vi "Accelerometer Display.vi"(1 "Accel Range":T2, 2 "Mode":enum8{"Start", "Run", "Finish"}(ring)) -> (0 "Distances":cluster{"X":dbl, "Y":dbl, "Z":dbl})   [LabVIEW 2014]
uses:
  <vilib>/Rock Robotics/WPI/Accelerometer/WPI_AccelerometerRange.ctl
  <vilib>/Rock Robotics/WPI/Accelerometer/InternalAccelerometer/WPI_AccelerometerInternalOpen.vi
  <vilib>/Analysis/NI_AALPro.lvlib
panel:
  out "Y Distance 2":dbl(graph)
  out "Z Distance":dbl(graph)
  out "Y Distance":dbl(graph)
  out "Waveform Chart":T1(graph)
  out "Z Acceleration":dbl
  out "Y Acceleration":dbl
  out "X Acceleration":dbl
  # "Set these inputs before running."
  # "Output information"
  # "This uses the internal accelerometer built into the roboRIO.  No wiring is necessary."
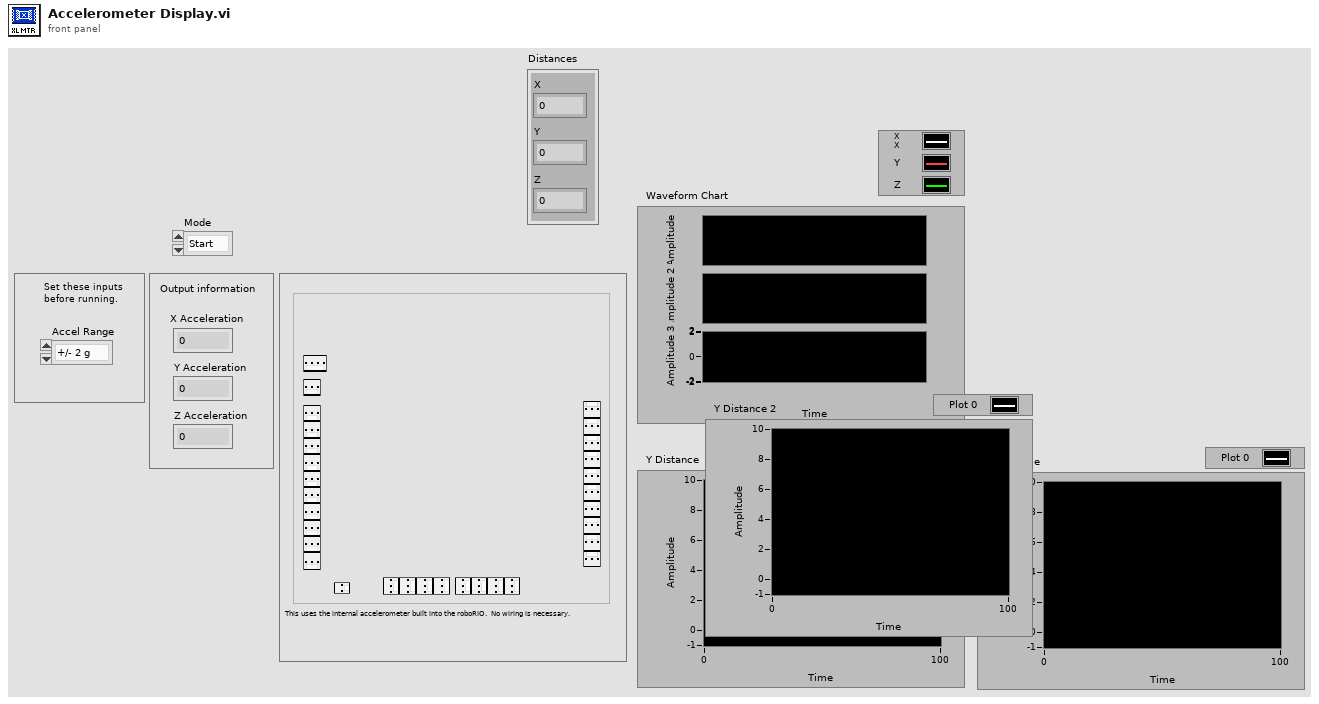
[diagram p1: front panel]
types:
  T1 = cluster{"X-Axis":dbl, "Y-Axis":dbl, "Z-Axis":dbl}
  T2 = typedef "WPI_AccelerometerRange.ctl" = enum16{"+/- 2 g", "+/- 4 g", "+/- 8 g"}
  T3 = typedef "WPI_AccelerometerDevRef.ctl" = cluster{"DevStatus":errorcluster, "Controller":T4, "Scaling":T5, "Analog Channels":T6, "I2C Bus":T8, "SPI Bus":T9, "Accel Range":T10, "ADXL345 Axes":T11, "Handle":i32, "Device Address":u8, "Accel Type":enum16{"Analog", "ADXL345 I2C", "ADXL345 SPI", "Internal"}}
  T4 = typedef "FPGA_TypedefAnalogModule.ctl" = enum16{"Controller 1"}
  T5 = typedef "WPI_AccelerometerScaling.ctl" = cluster{"Gain (VoltsPerG)":dbl, "Center Voltage":dbl}
  T6 = typedef "WPI_AccelerometerAnalogChannels.ctl" = cluster{"X-Axis":T7, "Y-Axis":T7, "Z-Axis":T7}
  T7 = typedef "FPGA_AIChannel.ctl" = enum8{"AI 0", "AI 1", "AI 2", "AI 3", "AI MXP 0", "AI MXP 1", "AI MXP 2", "AI MXP 3", "Invalid"}
  T8 = typedef "i2c_bus.ctl" = enum16{"I2C On-Board", "I2C MXP", "Invalid"}
  T9 = typedef "spi_bus.ctl" = enum16{"SPI On-Board, CS0", "SPI On-Board, CS1", "SPI On-Board, CS2", "SPI On-Board, CS3", "SPI MXP", "Invalid"}
  T10 = typedef "ADXL345 Range.ctl" = u8
  T11 = typedef "WPI_AccelerometerADXL345 Axes.ctl" = cluster{"X-Axis":bool, "Y-Axis":bool, "Z-Axis":bool}
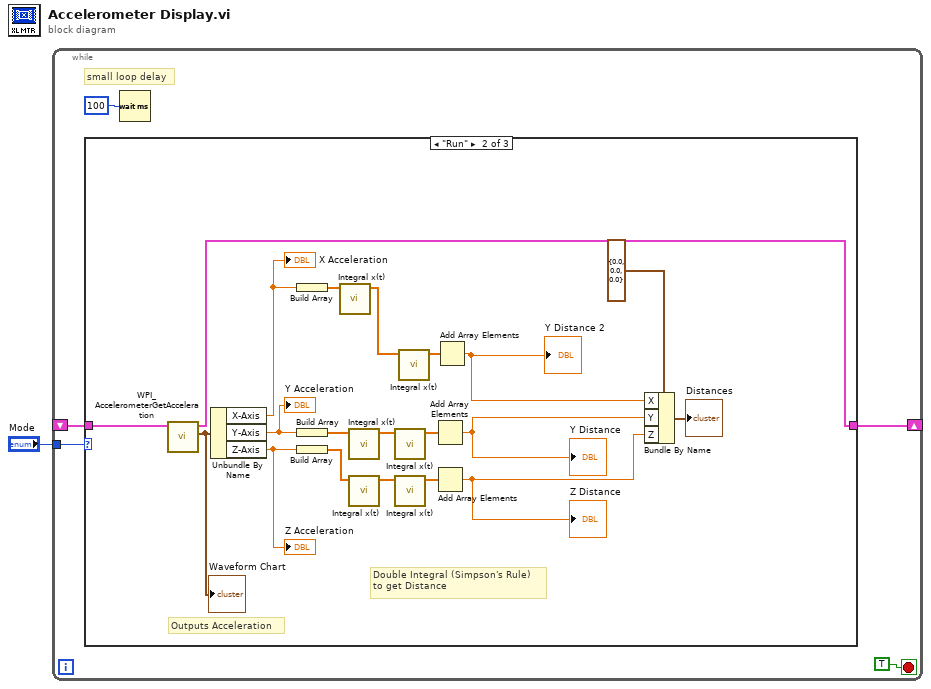
[diagram p0: block diagram]
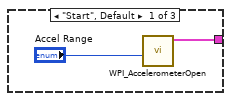
[diagram p2: hidden frame]
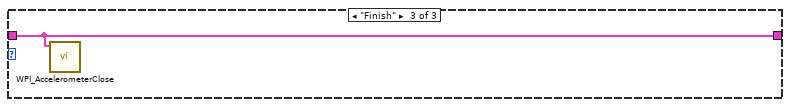
[diagram p3: hidden frame]
diagram:
  n1 = while {
    tunnel: "Mode" -> [w6]
    shift-right: [w4] -> _
    shift-left: _ -> [w3]
    stop <- TRUE stop-if-true
    # "small loop delay"
    n2 = case shown="\"Run\"" w6 {
      tunnel: [w7 w18 w29] -> w4
      tunnel: w3 -> [_ w28 w29]
      frame "Start", Default {
        n3 = call-poly <vilib>:"WPI_AccelerometerOpen.vi"("Accel Range"="Accel Range") -> ("AccelerometerDevRef"=w7:T3)  [unwired: 9 in, 1 out]
      }
      frame "Run" {
        # "Double Integral (Simpson's Rule)\nto get Distance"
        # "Outputs Acceleration"
        n4 = call <vilib>:"WPI_AccelerometerGetAcceleration.vi"("AccelerometerDevRef"=w28) -> ("Accelerations"=w27:T1, "AccelerometerDevRef"=w18:T3)  [unwired: 8 in, 1 out]
        "Waveform Chart" <- w27
        n5 = Unbundle By Name(w27) -> ("X-Axis"=w26:dbl, "Y-Axis"=w23:dbl, "Z-Axis"=w24:dbl)
        "X Acceleration" <- w26
        "Y Acceleration" <- w23
        "Z Acceleration" <- w24
        n6 = Build Array(w26) -> (w25:dbl[])
        n7 = Build Array(w23) -> (w22:dbl[])
        n8 = Build Array(w24) -> (w21:dbl[])
        n9 = call <vilib>:"Integral x(t).vi"("X"=w25) -> ("Integral X"=w11:dbl[])  [unwired: 9 in, 1 out]
        n10 = call <vilib>:"Integral x(t).vi"("X"=w22) -> ("Integral X"=w20:dbl[])  [unwired: 9 in, 1 out]
        n11 = call <vilib>:"Integral x(t).vi"("X"=w21) -> ("Integral X"=w19:dbl[])  [unwired: 9 in, 1 out]
        n12 = call <vilib>:"Integral x(t).vi"("X"=w20) -> ("Integral X"=w14:dbl[])  [unwired: 9 in, 1 out]
        n13 = call <vilib>:"Integral x(t).vi"("X"=w19) -> ("Integral X"=w15:dbl[])  [unwired: 9 in, 1 out]
        n14 = call <vilib>:"Integral x(t).vi"("X"=w11) -> ("Integral X"=w10:dbl[])  [unwired: 9 in, 1 out]
        n15 = Add Array Elements(numeric array=w14) -> (sum=w12:dbl)
        "Y Distance" <- w12
        n16 = Add Array Elements(numeric array=w15) -> (sum=w13:dbl)
        "Z Distance" <- w13
        n17 = Add Array Elements(numeric array=w10) -> (sum=w9:dbl)
        "Y Distance 2" <- w9
        n18 = Bundle By Name(cluster=cluster{"X":dbl, "Y":dbl, "Z":dbl} {"X"=0.0, "Y"=0.0, "Z"=0.0} ("Distances"), "X"=w9, "Y"=w12, "Z"=w13) -> (→"Distances":cluster{"X":dbl, "Y":dbl, "Z":dbl})
      }
      frame "Finish" {
        n19 = call <vilib>:"WPI_AccelerometerClose.vi"("AccelerometerDevRef"=w29) -> ()  [unwired: 10 in, 1 out]
      }
    }
    n20 = Wait (ms)(milliseconds to wait=u32 100) -> ()  [unwired: 1 out]
  }
